vi "禹山浊度_获取温度和测量值.vi"(8 "error in (no error)":errorcluster caption="错误输入（无错误）", 11 "MB session in":refnum<class "MB_Master.lvclass">) -> (0 "error out":errorcluster caption="错误输出", 2 "输出值":cluster{"温度测量值":sgl, "浊度":sgl}, 3 "MB session out":refnum<class "MB_Master.lvclass">)   [LabVIEW 2016, in "斯坦道多参数.lvlib"]
uses:
  <vilib>/Plasmionique/MB Master/MB_Master/MB_Master.lvclass
  <vilib>/Plasmionique/MB Master/MB Master.lvlib
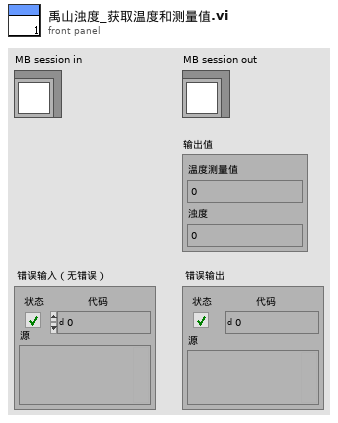
[diagram p1: front panel]
types:
  T1 = cluster{"pH":u32, "DO":u32, "Cond":u32, "Turb":u32, "叶绿素a":u32, "藻密度":u32, "ORP":u32, "COD":u32, "氯化物":u32, "氨氮":u32, "水中油":u32}
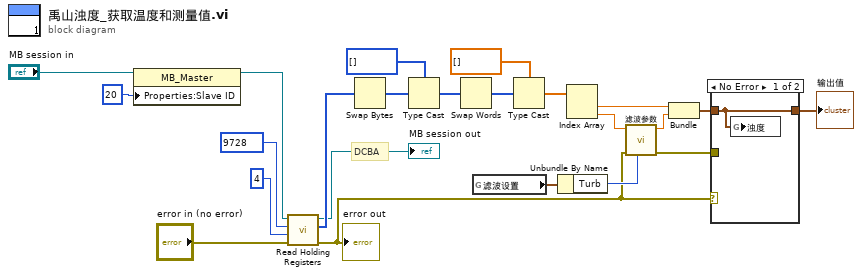
[diagram p0: block diagram]
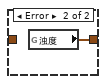
[diagram p2: hidden frame]
diagram:
  # "DCBA"
  n1 = property class="MB_Master"(reference="MB session in", "Properties:Slave ID"=u16 20 ("y")) -> (reference out=w15:refnum<class "MB_Master.lvclass">)  [unwired: 1 in, 1 out]
  n2 = call <vilib>:"Read Holding Registers.vi"("error in (no error)"="error in (no error)", "quantity"=u16 4, "starting address"=u16 9728, "MB session in"=w15) -> ("error out"=w2:errorcluster, "Registers"=w13:u16[], "MB session out"=→"MB session out":refnum<class "MB_Master.lvclass">)  [unwired: 5 in]
  "error out" <- w2
  n3 = Swap Bytes(anything=w13) -> (byte swapped=w12:u16[])
  n4 = Type Cast(type=u32[] [] ("数组 2"), x=w12) -> (*(type *) &x=w19:u32[])
  n5 = Swap Words(1:w19) -> (0:w21:u32[])
  n6 = global read "断电保存变量.vi" "滤波设置"() -> (w5:T1)
  n7 = Type Cast(type=sgl[] [] ("数组 2"), x=w21) -> (*(type *) &x=w17:sgl[])
  n8 = Unbundle By Name(w5) -> ("Turb"=w4:u32)
  n9 = Index Array(array=w17) -> (element #1=w11:sgl, element #2=w7:sgl)  [unwired: 2 in]
  n10 = call "滤波参数.vi"("滤波次数"=w4, "error in (no error)"=w2, "x"=w7) -> ("error out"=w1:errorcluster, "mode"=w6:dbl)  [unwired: 7 in]
  n11 = Bundle("数值"=w11, "mode"=w6) -> (w10:cluster{"数值":sgl, "mode":dbl})  [unwired: 1 in]
  n12 = case shown="No Error" w2 {
    tunnel: w10 -> [w24 _]
    tunnel: [w24 w25] -> w3
    tunnel: w1 -> [_ _]
    frame No Error {
      n13 = global write "禹山过程全局变量.vi" "浊度"(w24) -> ()
    }
    frame Error {
      n14 = global read "禹山过程全局变量.vi" "浊度"() -> (w25:cluster{"温度测量值":sgl, "浊度测量值":sgl})
    }
  }
  "输出值" <- w3
